vi "ShoulderTeleop.vi"(4 "CmdDownDec":bool, 6 "CmdUpInc":bool, 7 "CmdStop":bool, 8 "CmdCalcSpeaker":bool, 9 "CmdSpeaker":bool, 10 "CmdAmp":bool, 11 "CmdRest":bool) -> ()   [LabVIEW 2023]
doc: "Makes sure the actual position of the arm is within 5 degrees of the setpoint/target"
uses:
  <vilib>/Rock Robotics/WPI/ThirdParty/JAS_Junk/TrajLib/Trajectory_Library.lvlib
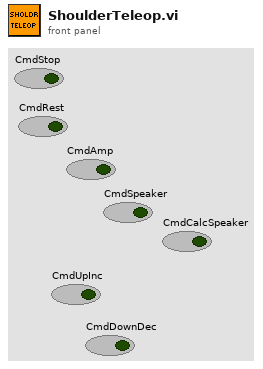
[diagram p1: front panel]
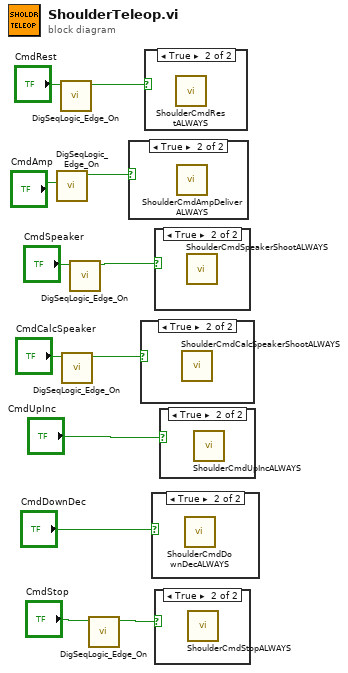
[diagram p0: block diagram]
diagram:
  n1 = call <vilib>:"DigSeqLogic_Edge_On.vi"("Input"="CmdAmp") -> ("On Edge"=w12:bool)  [unwired: 10 in]
  n2 = call <vilib>:"DigSeqLogic_Edge_On.vi"("Input"="CmdRest") -> ("On Edge"=w10:bool)  [unwired: 10 in]
  n3 = call <vilib>:"DigSeqLogic_Edge_On.vi"("Input"="CmdCalcSpeaker") -> ("On Edge"=w11:bool)  [unwired: 10 in]
  n4 = call <vilib>:"DigSeqLogic_Edge_On.vi"("Input"="CmdSpeaker") -> ("On Edge"=w9:bool)  [unwired: 10 in]
  n5 = call <vilib>:"DigSeqLogic_Edge_On.vi"("Input"="CmdStop") -> ("On Edge"=w2:bool)  [unwired: 10 in]
  n6 = case shown="True" w12 {
    frame False {
    }
    frame True {
      n7 = call "ShoulderCmdAmpDeliverALWAYS.vi"() -> ()  [unwired: 11 in, 1 out]
    }
  }
  n8 = case shown="True" w11 {
    frame False {
    }
    frame True {
      n9 = call "ShoulderCmdCalcSpeakerShootALWAYS.vi"() -> ()  [unwired: 11 in, 1 out]
    }
  }
  n10 = case shown="True" w10 {
    frame False {
    }
    frame True {
      n11 = call "ShoulderCmdRestALWAYS.vi"() -> ()  [unwired: 11 in, 1 out]
    }
  }
  n12 = case shown="True" "CmdDownDec" {
    frame False {
    }
    frame True {
      n13 = call "ShoulderCmdDownDecALWAYS.vi"() -> ()  [unwired: 11 in, 1 out]
    }
  }
  n14 = case shown="True" w9 {
    frame False {
    }
    frame True {
      n15 = call "ShoulderCmdSpeakerShootALWAYS.vi"() -> ()  [unwired: 11 in, 1 out]
    }
  }
  n16 = case shown="True" w2 {
    frame False {
    }
    frame True {
      n17 = call "ShoulderCmdStopALWAYS.vi"() -> ()  [unwired: 11 in, 1 out]
    }
  }
  n18 = case shown="True" "CmdUpInc" {
    frame False {
    }
    frame True {
      n19 = call "ShoulderCmdUpIncALWAYS.vi"() -> ()  [unwired: 11 in, 1 out]
    }
  }
